vi "Get Terminal from Node By Name.vi"(8 "error in (no error)":errorcluster, 10 "Terminal Name":string, 11 "Node":refnum<vi>) -> (0 "error out":errorcluster, 1 "Found?":bool, 2 "Terminal":refnum<vi>, 3 "Node out":refnum<vi>)   [LabVIEW 2020, in "JKI State Machine API.lvlib" / "JKI SM.lvclass"]
uses:
  JKI SM.lvclass
panel:
  out "Array":string[](array[string])
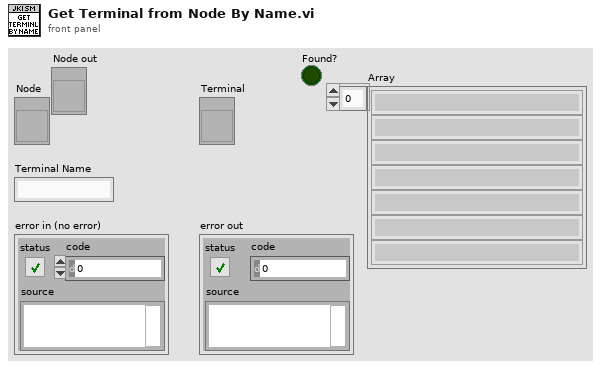
[diagram p1: front panel]
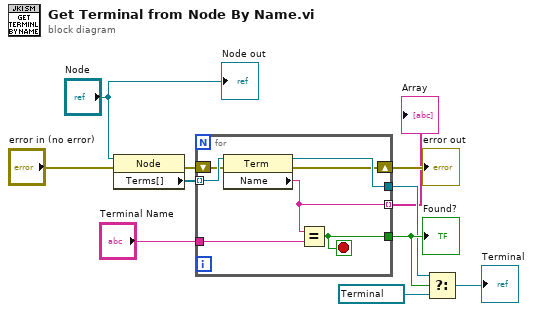
[diagram p0: block diagram]
diagram:
  n1 = property class="Node"(reference="Node", error in="error in (no error)") -> (error out=w9:errorcluster, "Terms[]"=w11:refnum<vi>[])  [unwired: 1 out]
  n2 = for {
    tunnel: w11 -> [w18] mode=indexing
    tunnel: "Terminal Name" -> [w17]
    tunnel: [w16] -> w5
    shift-right: [w14] -> w8
    shift-left: w9 -> [w15]
    tunnel: [w12] -> w6
    tunnel: [w13] -> w1 mode=indexing
    stop <- w12 stop-if-true
    n3 = property class="Term"(reference=w18, error in=w15) -> (reference out=w16:refnum<vi>, error out=w14:errorcluster, "Name"=w13:string)
    n4 = Equal?(x=w13, y=w17) -> (x = y?=w12:bool)
  }
  "error out" <- w8
  "Found?" <- w6
  "Array" <- w1
  n5 = Select(t=w5, s=w6, f=refnum<vi> refnum) -> (s? t:f=→"Terminal":refnum<vi>)
  "Node out" <- "Node"
